vi "Yokogawa GX20 Acquire Continuous Measurement Data Example RS422.vi"() -> ()   [LabVIEW 2020]
doc: "This example shows how to configure multiple channels and acquire measurement data from multiple channels."
uses:
  <instrlib>/Yokogawa GX Series/Public/Data/Read Measurement Data (Analog NChan).vi
  <instrlib>/Yokogawa GX Series/Yokogawa GX Series.lvlib
panel:
  in  "User ID (\"\")":string
  in  "Password (\"\")":string
  in  "User Name (\"\")":string
  in  "Serial Configuration":T1={"Baud Rate"=9600, "Parity"=2, "Data Bits"=8, "Flow Control"=0} {"Flow Control" items=["None", "XON/XOFF", "RTS/CTS", "XON/XOFF & RTS/CTS"]; "Data Bits" items=["7"=7, "8"=8]; "Parity" items=["None", "Odd", "Even"]; "Baud Rate" items=["1200"=1200, "2400"=2400, "4800"=4800, "9600"=9600, "19200"=19200, "38400"=38400, "57600"=57600, "115200"=115200]}
  out "Ch":string[](array[string])
  out "Unit":string[](array[string])
  out "Data":dbl[](array[numeric]) format="%#_5f"
  in  "Interval (1000)":u32=1000 min=25
  out "Date Time":timestamp=timestamp(3345116400 s since 1904-01-01) format="%<%H:%M:%S%3u\n%x>T"
  in  "End Channel (0010)":string="0010"
  in  "Start Channel (0001)":string="0001"
  in  "VISA resource name":refnum<visa-resource-name>
  in  "Stop":bool
  out "Chart":dbl[][](graph)
  # "(c) 2013-2018 Yokogawa Electric Corporation.  ALL RIGHTS RESERVED."
  # "GX/GP/GM PAPERLESS RECORDER"
  # "ms"
  # "To execute this example, do below.\n1) Attach AI module to GX/GP/GM.\n2) Do Reconfiguring the GX/GP/GM (See User's Manual 1.24.2)\n3) Run this VI with valid VISA resource name (ex: \"COM1\")"
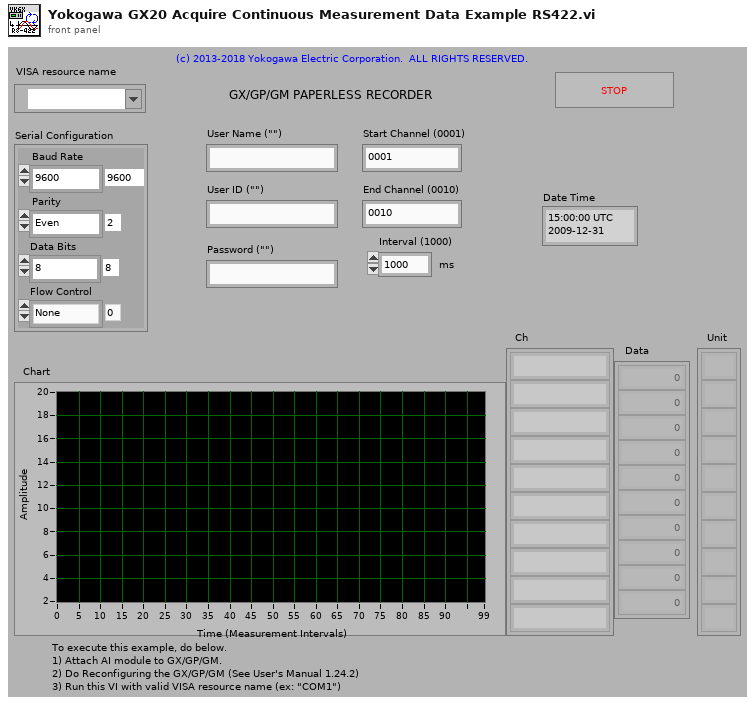
[diagram p1: front panel]
types:
  T1 = cluster{"Baud Rate":u32, "Parity":u16, "Data Bits":u16, "Flow Control":u16}
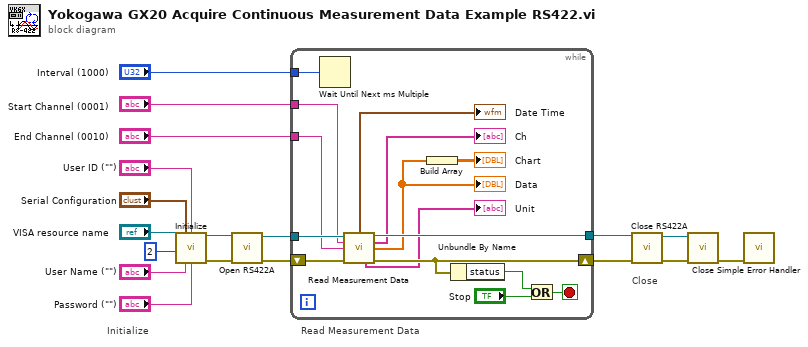
[diagram p0: block diagram]
diagram:
  # "Read Measurement Data"
  # "Close"
  # "Initialize"
  n1 = call <instrlib>:"Initialize.vi"("VISA resource name IN"="VISA resource name", "Serial Configuration"="Serial Configuration", "User ID (\"\")"="User ID (\"\")", "Serial Auth Type (0: Not Auth)"=2, "User Name (\"admin\")"="User Name (\"\")", "Password (\"\")"="Password (\"\")") -> ("VISA resource name out"=w12:refnum<visa-resource-name>, "error out"=w13:errorcluster)  [unwired: 8 in]
  n2 = call <instrlib>:"Open RS422A.vi"("error in (no error)"=w13, "VISA resource name"=w12) -> ("error out"=w5:errorcluster, "VISA resource name out"=w11:refnum<visa-resource-name>)  [unwired: 8 in]
  n3 = while {
    shift-left: w5 -> [w28]
    shift-right: [w30] -> w7
    tunnel: [w29] -> w8
    tunnel: w11 -> [w27]
    tunnel: "Interval (1000)" -> [w25]
    tunnel: "Start Channel (0001)" -> [w24]
    tunnel: "End Channel (0010)" -> [w23]
    stop <- w32 stop-if-true
    n4 = Wait Until Next ms Multiple(millisecond multiple=w25) -> ()  [unwired: 1 out]
    n5 = call-poly <instrlib>:"Read Measurement Data.vi"("VISA resource name"=w27, "Start Channel (1)"=w24, "End Channel (1)"=w23, "error in (no error)"=w28) -> ("Date Time"=→"Date Time":timestamp, "VISA resource name out"=w29:refnum<visa-resource-name>, "Channel"=→"Ch":string[], "Data"=w22:dbl[], "Unit"=→"Unit":string[], "error out"=w30:errorcluster)  [unwired: 1 in, 5 out]
    "Data" <- w22
    n6 = Build Array(w22) -> (→"Chart":dbl[][])
    n7 = Unbundle By Name(w30) -> ("status"=w31:bool)
    n8 = Or(x=w31, y="Stop") -> (x .or. y?=w32:bool)
  }
  n9 = call <instrlib>:"Close RS422A.vi"("error in (no error)"=w7, "VISA resource name"=w8) -> ("error out"=w10:errorcluster, "VISA resource name out"=w9:refnum<visa-resource-name>)  [unwired: 8 in]
  n10 = call <instrlib>:"Close.vi"("error in (no error)"=w10, "VISA resource name"=w9) -> ("error out"=w18:errorcluster)  [unwired: 9 out]
  n11 = call <vilib>:"Simple Error Handler.vi"("error in (no error)"=w18) -> ()  [unwired: 1 in, 8 out]
